vi "FTW-ActorConfig-FormatExtendedPublishers.vi"(0 "FTW Config String In":string="{}", 5 "Publisher Names":string[](array[string]), 7 "Publisher Addresses":string[](array[string]), 11 "error in":errorcluster) -> (4 "FTW Config String":string, 15 "error out":errorcluster)   [LabVIEW 2015]
uses:
  container/FTW-Container.lvclass
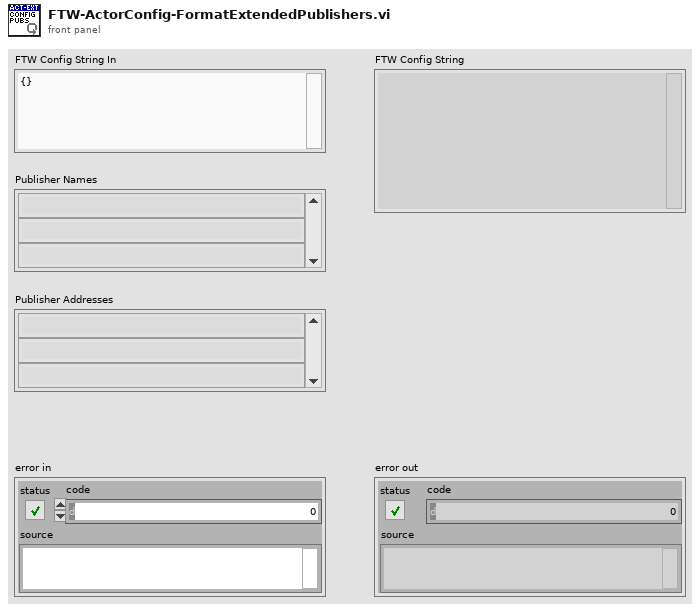
[diagram p1: front panel]
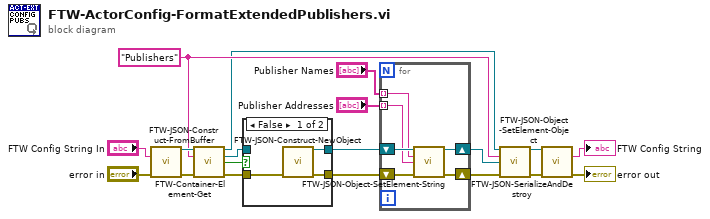
[diagram p0: block diagram]
diagram:
  w6 = "Publishers" ("Element Name")
  n1 = call "FTW-JSON-Construct-FromBuffer.vi"("JSON String (UTF-8)"="FTW Config String In", "error in"="error in") -> ("JSON"=w17:refnum<class "FTW-Container.lvclass">, "error out"=w16:errorcluster)  [unwired: 12 in]
  n2 = call "FTW-Container-Element-Get.vi"("FTW-Container In"=w17, "Element Name"=w6, "error in"=w16) -> ("FTW-Container Out"=w5:refnum<class "FTW-Container.lvclass">, "Element Out"=w14:refnum<class "FTW-Container.lvclass">, "Found"=w15:bool, "error out"=w13:errorcluster)  [unwired: 9 in]
  n3 = case shown="False" w15 {
    tunnel: w14 -> [_ w24]
    tunnel: w13 -> [w22 w23]
    tunnel: [w21 w24] -> w11
    tunnel: [w20 w23] -> w12
    frame False {
      n4 = call "FTW-JSON-Construct-NewObject.vi"("error in"=w22) -> ("JSON"=w21:refnum<class "FTW-Container.lvclass">, "error out"=w20:errorcluster)  [unwired: 13 in]
    }
    frame True {
    }
  }
  n5 = for {
    tunnel: "Publisher Names" -> [w28] mode=indexing
    shift-right: [w27] -> w9
    shift-left: w12 -> [w30]
    shift-right: [w26] -> w8
    shift-left: w11 -> [w29]
    tunnel: "Publisher Addresses" -> [w25] mode=indexing
    n6 = call "FTW-JSON-Object-SetElement-String.vi"("JSON"=w29, "Key"=w28, "Value"=w25, "error in"=w30) -> ("JSON out"=w26:refnum<class "FTW-Container.lvclass">, "error out"=w27:errorcluster)  [unwired: 10 in]
  }
  n7 = call "FTW-JSON-Object-SetElement-Object.vi"("JSON Object"=w5, "Key"=w6, "JSON Sub-Object"=w8, "error in"=w9) -> ("JSON Root Object"=w3:refnum<class "FTW-Container.lvclass">, "error out"=w4:errorcluster)  [unwired: 10 in]
  n8 = call "FTW-JSON-SerializeAndDestroy.vi"("JSON"=w3, "error in"=w4) -> ("JSON String (UTF-8)"=→"FTW Config String":string, "error out"=→"error out":errorcluster)  [unwired: 12 in]
